vi "Cvrt Strain Gauge Reading.vi"(6 "Vinit (0.0)":dbl, 11 "Strain in":refnum<class "Strain.lvclass">) -> (2 "Strain":sgl)   [LabVIEW 2012, in "Measurement Channels.lvlib" / "Strain.lvclass"]
uses:
  Strain.lvclass
  Strain.lvclass/Strain.ctl
  <vilib>/Utility/TradDaqScaling.llb/Convert Strain Gauge Reading (scaler).vi
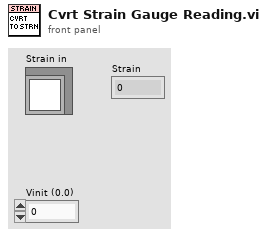
[diagram p1: front panel]
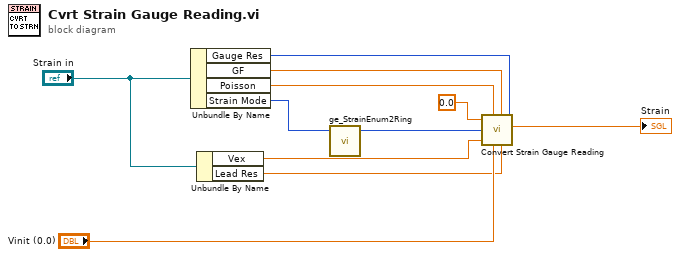
[diagram p0: block diagram]
diagram:
  n1 = Unbundle By Name("Strain in") -> ("Gauge Res"=w6:i32, "GF"=w5:dbl, "Poisson"=w4:dbl, "Strain Mode"=w3:u16)
  n2 = Unbundle By Name("Strain in") -> ("Vex"=w2:dbl, "Lead Res"=w1:dbl)
  n3 = call "ge_StrainEnum2Ring.vi"("Bridge Type"=w3) -> ("Bridge Config Ring"=w8:u16)  [unwired: 4 in]
  n4 = call-poly <vilib>:"Convert Strain Gauge Reading.vi"("Vsg (0.0)"=sgl 0.0 ("v (0.0)"), "v (0.0)"=w4, "Bridge Configuration\n(3:Half Bridge II)"=w8, "Vex (3.33)"=w2, "Vinit (0.0)"="Vinit (0.0)", "GF (2.0)"=w5, "Rg (120)"=w6, "Rl (0.0)"=w1) -> ("Strain"=→"Strain":sgl)  [unwired: 2 in]
